vi "Set Initialization Data - Maes-Acq.vi"(8 "error in":errorcluster, 11 "Maestro Control in":refnum<class "Maestro Control.lvclass">) -> (0 "error out":errorcluster, 3 "Maestro Control out":refnum<class "Maestro Control.lvclass">)   [LabVIEW 2021, in "Maestro Control.lvclass"]
doc: "Sets the initialization data of a statically linked subWorker."
uses:
  Maestro Control.lvclass
  C:/Program Files (x86)/National Instruments/LabVIEW 2021/vi.lib/addons/_Workers/Library/Classes/Worker/Worker.lvclass
  Maestro Acq/Initialization Data.ctl
  <vilib>/addons/_Workers/Library/Classes/Message Queue/Message Queue.lvclass
  Maestro Acq/Hardware Maestro Config.ctl
  <vilib>/addons/_Workers/Library/Classes/Worker/Worker.lvclass/Worker.ctl
  Maestro Control.lvclass/Maestro Control.ctl
  Maestro Acq/Maestro Acq.lvclass
  <vilib>/addons/_Workers/Library/Classes/Worker/Worker.lvclass
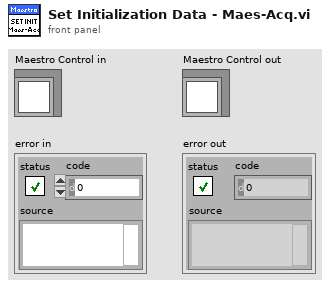
[diagram p1: front panel]
types:
  T1 = typedef "Maestro Acq.lvclass/Initialization Data.ctl" = cluster{"String":string, "Maestro Ctrl Queue":refnum<class "Message Queue.lvclass">, "Hardware Maestro Config":T2, "Data Queue":refnum<queue>, "Data Notifier":refnum<notifier>}
  T2 = typedef "Maestro Acq.lvclass/Hardware Maestro Config.ctl" = cluster{"Adress(ip)":string, "Port":i16, "Log File Base Path":path, "délai d'acq.(ms)":i32, "Activer les Stats":bool}
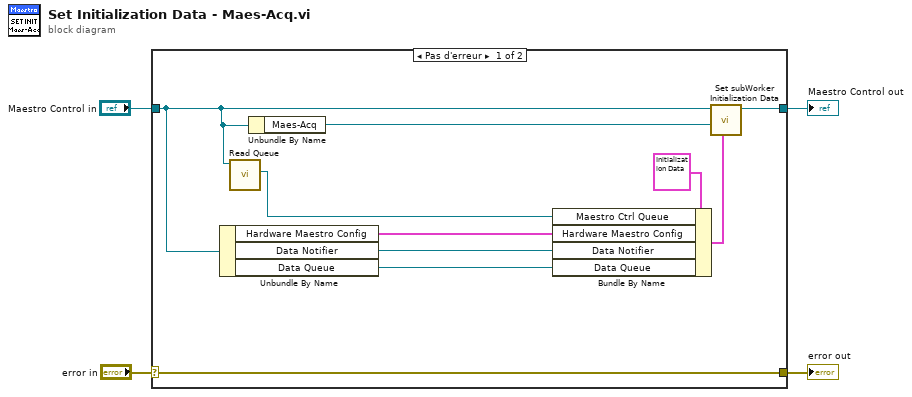
[diagram p0: block diagram]
diagram:
  n1 = case shown="Pas d'erreur" "error in" {
    selector: "error in" -> [w14 w16]
    tunnel: [w14 w16] -> w3
    tunnel: [w13 w15] -> w2
    tunnel: "Maestro Control in" -> [w8 w15]
    frame No Error {
      n2 = Unbundle By Name(w8) -> ("Hardware Maestro Config"=w10:T2, "Data Notifier"=w6:refnum<notifier>, "Data Queue"=w5:refnum<queue>)
      n3 = call <vilib>:"Read Queue.vi"("Worker"=w8) -> ("Message Queue out"=w7:refnum<class "Message Queue.lvclass">)  [unwired: 9 in, 1 out]
      n4 = Unbundle By Name(w8) -> ("Maes-Acq"=w9:refnum<class "Maestro Acq.lvclass">)
      n5 = Bundle By Name(cluster=T1 {"String"="", "Maestro Ctrl Queue"=refnum, "Hardware Maestro Config"={"Adress(ip)"="", "Port"=0, "Log File Base Path"=path "", "délai d'acq.(ms)"=0, "Activer les Stats"=FALSE}, "Data Queue"=refnum, "Data Notifier"=refnum} ("Initialization Data"), "Maestro Ctrl Queue"=w7, "Hardware Maestro Config"=w10, "Data Notifier"=w6, "Data Queue"=w5) -> (w11:T1)
      n6 = call-dynamic "Set subWorker Initialization Data.vi"("Initialization Data"=w11, "subWorker"=w9, "Worker"=w8) -> ("Worker out"=w13:refnum<class "Maestro Control.lvclass">)  [unwired: 8 in]
    }
    frame Error {
    }
  }
  "error out" <- w3
  "Maestro Control out" <- w2
